vi "SUB_Writelog.vi"(2 "Pass/Fail":string) -> ()   [LabVIEW 2011]
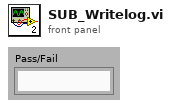
[diagram p1: front panel]
types:
  T1 = enum32{"invalid app kind", "Development System", "Run Time System", "Student Edition", "Embedded LabVIEW", "Evaluation", "Custom"}
  T2 = enum16{"open", "replace", "create", "open or create", "replace or create", "replace or create with confirmation"}
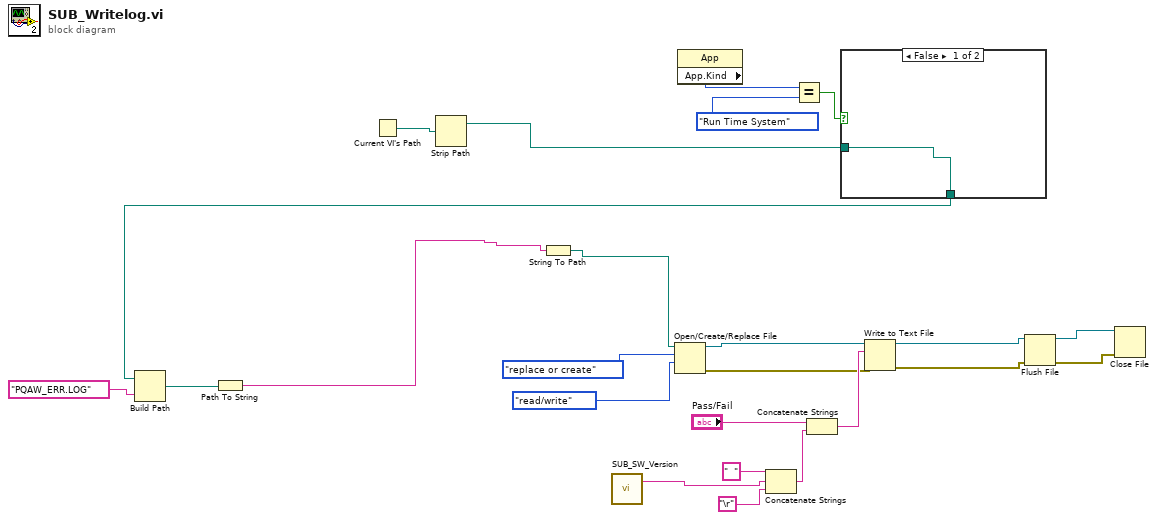
[diagram p0: block diagram]
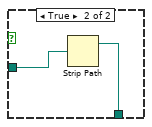
[diagram p2: hidden frame]
diagram:
  n1 = Current VI's Path() -> (path=w19:path)
  n2 = Strip Path(path=w19) -> (stripped path=w15:path)  [unwired: 1 out]
  n3 = call "SUB_SW_Version.vi"() -> ("Current Software Version"=w8:string)  [unwired: 3 in]
  n4 = property class="App"() -> ("App.Kind"=w18:T1)  [unwired: 2 in, 2 out]
  n5 = Concatenate Strings("  ", w8, "\r") -> (w5:string)
  n6 = Equal?(x=w18, y=T1."Run Time System" ("Application:Kind")) -> (x = y?=w16:bool)
  n7 = Concatenate Strings("Pass/Fail", w5) -> (w22:string)
  n8 = case shown="False" w16 {
    tunnel: w15 -> [w25 w27]
    tunnel: [w25 w26] -> w10
    frame False {
    }
    frame True {
      n9 = Strip Path(path=w27) -> (stripped path=w26:path)  [unwired: 1 out]
    }
  }
  n10 = Build Path(base path=w10, name or relative path="PQAW_ERR.LOG" ("string")) -> (appended path=w12:path)
  n11 = Path To String(path=w12) -> (string=w9:string)
  n12 = String To Path(string=w9) -> (path=w14:path)
  n13 = Open/Create/Replace File(file path (use dialog)=w14, operation (0:open)=T2."replace or create", access (0:read/write)=enum16{"read/write", "read-only", "write-only"}."read/write") -> (refnum out=w21:refnum<file>, error out=w13:errorcluster)  [unwired: 3 in, 1 out]
  n14 = Write to Text File(file (use dialog)=w21, text=w22, error in=w13) -> (refnum out=w4:refnum<file>, error out=w3:errorcluster)  [unwired: 1 in, 1 out]
  n15 = Flush File(refnum=w4, error in=w3) -> (refnum out=w2:refnum<file>, error out=w1:errorcluster)
  n16 = Close File(refnum=w2, error in=w1) -> ()  [unwired: 2 out]
